vi "fake lock-in module.vi"(9 "Master mailbox":T6, 11 "Module mailbox":T6) -> ()   [LabVIEW 2024, in "Lock-in module.lvlib"]
uses:
  Lock-in module.lvlib
  Messenger service/Data types/Mailbox address.ctl
  ctl/ACQ status.ctl
  <instrlib>/Zurich Instruments LabOne/Public/ziTypeHandle.ctl
  <instrlib>/Zurich Instruments LabOne/Public/Modules/ziTypeModHandle.ctl
  ctl/ACQ info.ctl
  ctl/Mode.ctl
  Messenger service/Data types/Module name.ctl
  ctl/MFLI_message for module.ctl
  ctl/MFLI_command enum.ctl
  ctl/ACQ parameters.ctl
  ctl/MFLI_parameter and value.ctl
  ctl/MFLI_node.ctl
  <instrlib>/Zurich Instruments LabOne/Public/Data/ziTypeDemodSampleSingle.ctl
  <instrlib>/Zurich Instruments LabOne/Zurich Instruments LabOne.lvlib
  Messenger service/MessengerLib.lvlib
panel:
  out "Mode":T1=enum."Point"
  out "ACQ  status":T2={"Lock-in Handle"={"handleValid"=FALSE, "Conn"=0, "Path Prefix"="", "Handle"=0, "Connected"=FALSE, "Clockbase(s)"=0.0}, "Address"="DEV", "ModuleHandles"=[], "Lock-in info"={"In50"=FALSE, "InAC"=FALSE, "InDiff"=FALSE, "Out50"=FALSE, "OutEN"=FALSE, "OutF[Hz]"=0.0, "OutA[V]"=0.0, "DemEN"=FALSE, "Const[ms]"=0.0, "Order[-]"=0, "Phase [°]"=0.0}} {"ModuleHandles"."ModHandle" format="0x%08x"; "ModuleHandles"."Conn" format="0x%08x"; "Lock-in Handle"."Handle" format="0x%08x"; "Lock-in Handle"."Conn" format="0x%08x"}
  out "Selected Device":string
  out "Initialized":bool
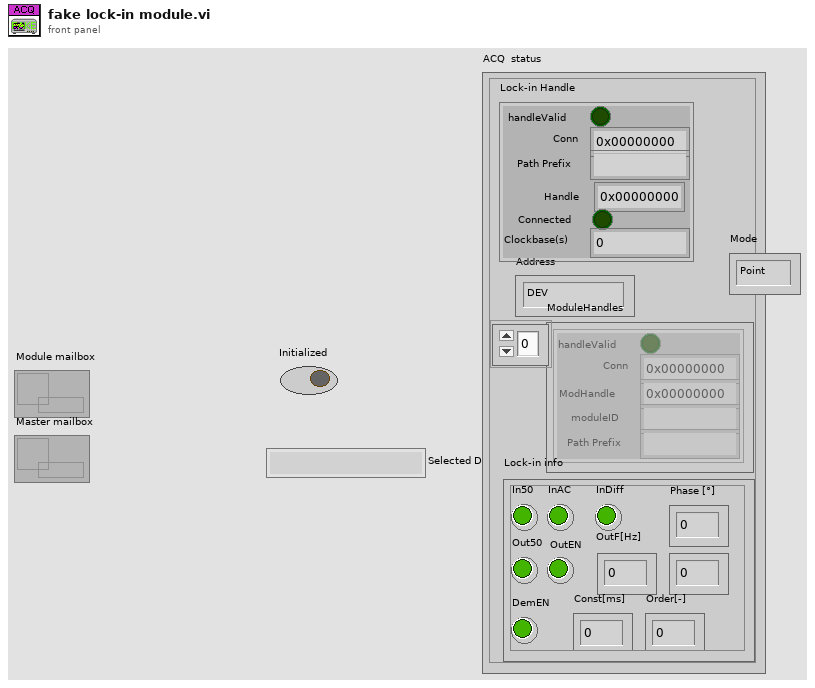
[diagram p1: front panel]
types:
  T1 = typedef "Lock-in module.lvlib/Mode.ctl" = enum16{"None", "Point", "Scope", "Both", "DAQ"}
  T2 = typedef "Lock-in module.lvlib/ACQ status.ctl" = cluster{"Lock-in Handle":T3, "Address":string, "ModuleHandles":T4[], "Lock-in info":T5}
  T3 = typedef "Zurich Instruments LabOne.lvlib/ziTypeHandle.ctl" = cluster{"handleValid":bool, "Conn":u64, "Path Prefix":string, "Handle":u64, "Connected":bool, "Clockbase(s)":dbl}
  T4 = typedef "Zurich Instruments LabOne.lvlib/ziTypeModHandle.ctl" = cluster{"handleValid":bool, "Conn":u64, "ModHandle":u64, "moduleID":string, "Path Prefix":string}
  T5 = typedef "Lock-in module.lvlib/ACQ info.ctl" = cluster{"In50":bool, "InAC":bool, "InDiff":bool, "Out50":bool, "OutEN":bool, "OutF[Hz]":dbl, "OutA[V]":dbl, "DemEN":bool, "Const[ms]":dbl, "Order[-]":i32, "Phase [°]":dbl}
  T6 = typedef "MessengerLib.lvlib/Mailbox address.ctl" = refnum<queue>
  T7 = typedef "Module name.ctl" = enum16{"Emty", "Magnet", "VTI", "Excitation", "Servo", "Acquisition", "Rotator", "Digitizer", "SMU2450", "Carousel", "Multimeter", "Tmp monitor", "Power monitor"}
  T8 = typedef "Lock-in module.lvlib/ACQ parameters.ctl" = cluster{"Filter order":dbl, "Time constant [ms]":dbl, "F_Mod [kHz]":dbl, "Amp_Mod [mV]":dbl, "Enable output":u16, "Phase [°]":dbl}
  T9 = typedef "Lock-in module.lvlib/MFLI_parameter and value.ctl" = cluster{"parameter":T10, "value":dbl}
  T10 = typedef "Lock-in module.lvlib/MFLI_node.ctl" = enum16{"None", "filter_order [-]", "filter_constant [ms]", "in_diff", "in_autorange", "in_imp50", "in_AC", "osc_freq [kHz]", "out_ampl [V]", "out_autorange", "out_imp50", "enable output", "enamble ampl", "scope_enable", "scope_rate", "scope_len", "scope_trigEn", "AuxOut_amplify", "Phase_deg", "AuxOut_select"}
  T11 = typedef "Zurich Instruments LabOne.lvlib/ziTypeDemodSampleSingle.ctl" = cluster{"Timestamps (ticks)":u64, "X (Vrms)":dbl, "Y (Vrms)":dbl, "Osc Phase (deg)":dbl, "Freq (Hz)":dbl, "DIO":u32, "AuxIn0 (V)":dbl, "AuxIn1 (V)":dbl, "Trigger":u32}
  T12 = typedef "Lock-in module.lvlib/MFLI_command enum.ctl" = enum16{"Initialize", "Update", "Set parameters", "Set module", "Set individual parameters", "Get point", "Get array", "Disconnect", "End", "Ignore"}
  T13 = typedef "Lock-in module.lvlib/MFLI_message for module.ctl" = cluster{"Command":T12, "Data":variant}
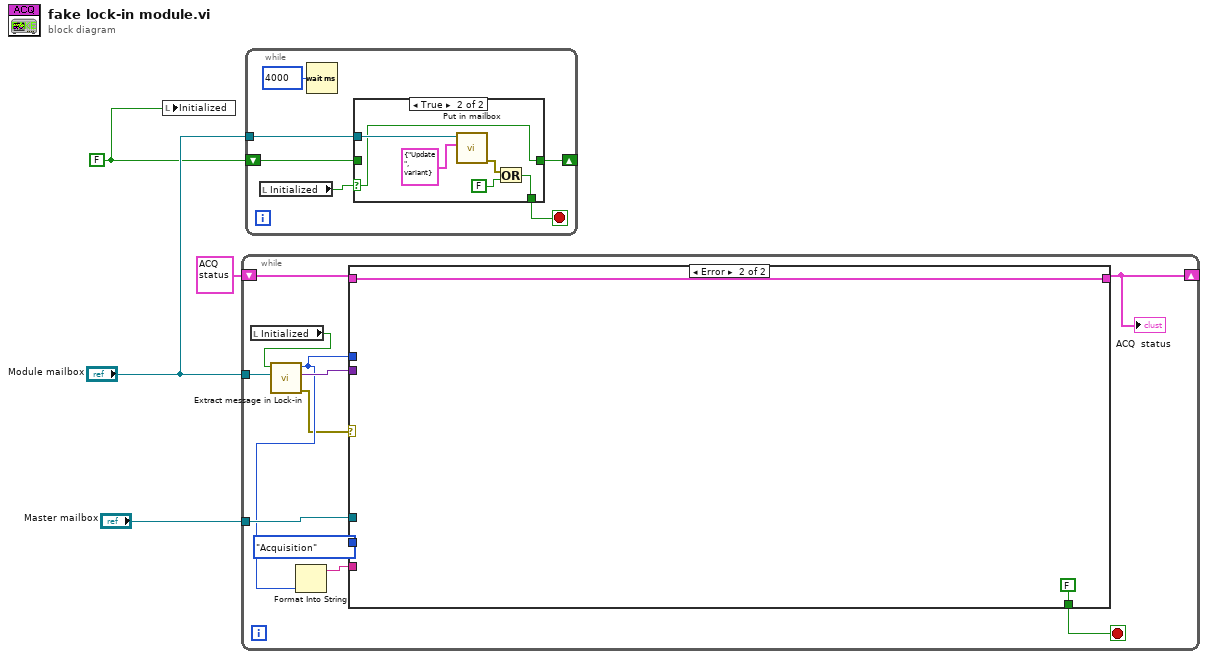
[diagram p0: block diagram]
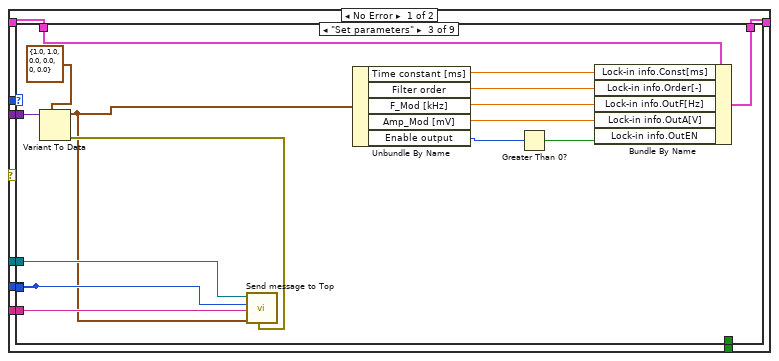
[diagram p2: hidden frame]
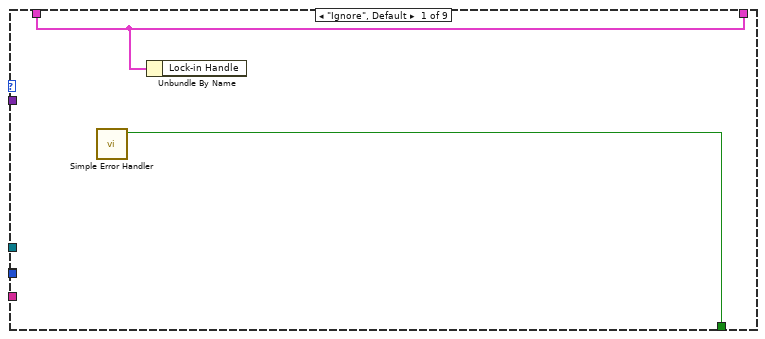
[diagram p3: hidden frame]
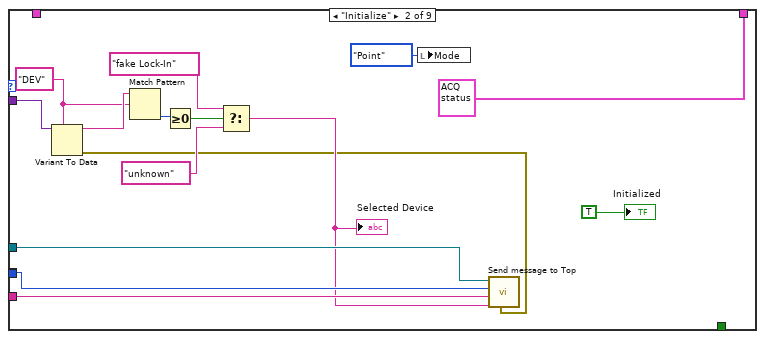
[diagram p4: hidden frame]
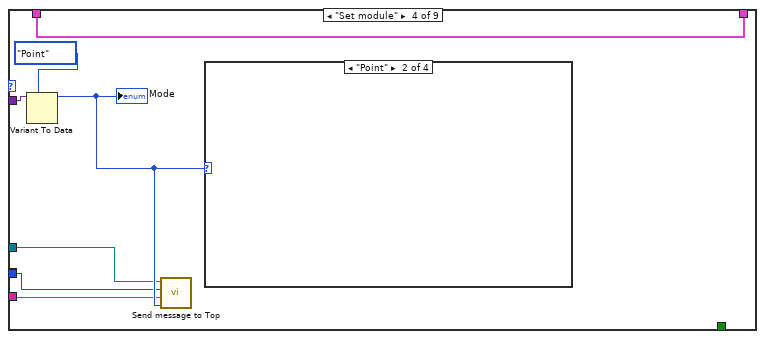
[diagram p5: hidden frame]
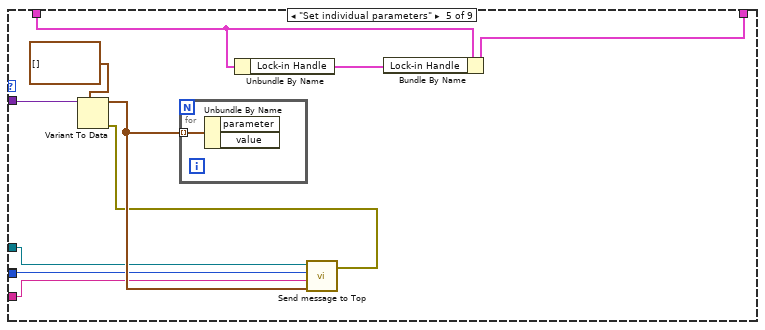
[diagram p9: hidden frame]
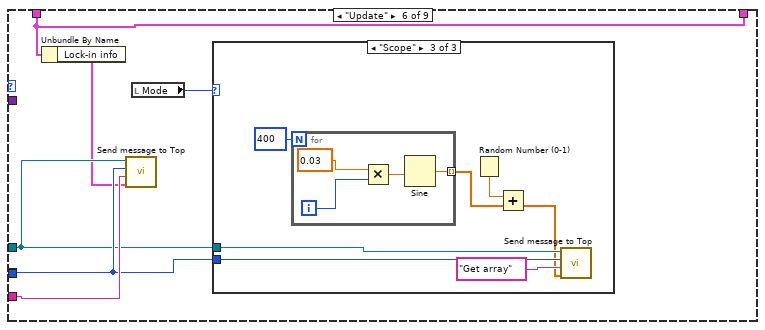
[diagram p10: hidden frame]
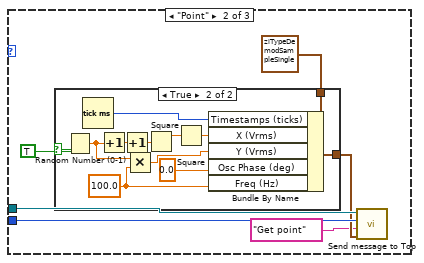
[diagram p12: hidden frame]
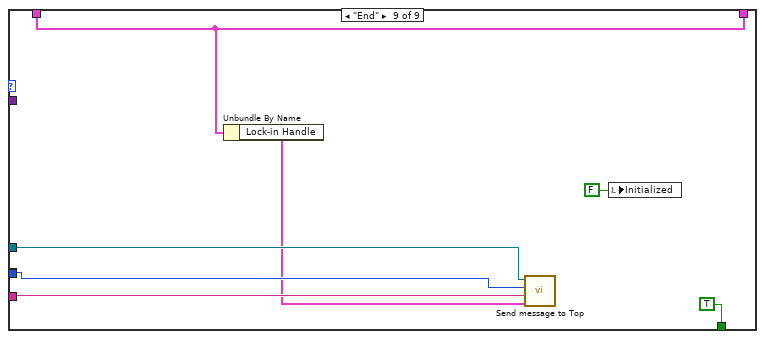
[diagram p16: hidden frame]
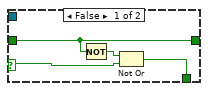
[diagram p17: hidden frame]
diagram:
  w1 = FALSE
  n1 = local write "Initialized"(w1) -> ()
  n2 = while {
    tunnel: "Module mailbox" -> [w15]
    tunnel: "Master mailbox" -> [w14]
    shift-right: [w11] -> _
    shift-left: T2 {"Lock-in Handle"={"handleValid"=FALSE, "Conn"=0, "Path Prefix"="", "Handle"=0, "Connected"=FALSE, "Clockbase(s)"=0.0}, "Address"="DEV", "ModuleHandles"=[], "Lock-in info"={"In50"=FALSE, "InAC"=FALSE, "InDiff"=FALSE, "Out50"=FALSE, "OutEN"=FALSE, "OutF[Hz]"=0.0, "OutA[V]"=0.0, "DemEN"=FALSE, "Const[ms]"=0.0, "Order[-]"=0, "Phase [°]"=0.0}} -> [w10]
    stop <- w12 stop-if-true
    n3 = local read "Initialized"() -> (w9:bool)
    n4 = call "Extract message in Lock-in.vi"("Module mailbox"=w15, "Initialized?"=w9) -> ("error out"=w5:errorcluster, "Data"=w13:variant, "Command out"=w7:T12)  [unwired: 7 in]
    n5 = Format Into String(w7) -> (resulting string=w8:string)  [unwired: 3 in, 1 out]
    n6 = case shown="Error" w5 {
      tunnel: w14 -> [w23 _]
      tunnel: w13 -> [w22 _]
      tunnel: [w21 FALSE ("error?")] -> w12
      tunnel: [w20 w119] -> w11
      tunnel: w10 -> [w19 w119]
      tunnel: w8 -> [w18 _]
      tunnel: w7 -> [w17 _]
      tunnel: Module_name."Acquisition" ("Module") -> [w16 _]
      frame No Error {
        n7 = case shown="\"Set parameters\"" w17 {
          tunnel: w23 -> [_ w39 w51 w56 w64 w76 _ _ w115]
          tunnel: w22 -> [_ w40 w55 w61 w72 _ _ _ _]
          tunnel: [w25 _ _ _ _ _ _ _ TRUE] -> w21
          tunnel: [w24 T2 {"Lock-in Handle"={"handleValid"=FALSE, "Conn"=0, "Path Prefix"="", "Handle"=0, "Connected"=FALSE, "Clockbase(s)"=0.0}, "Address"="DEV", "ModuleHandles"=[], "Lock-in info"={"In50"=FALSE, "InAC"=FALSE, "InDiff"=FALSE, "Out50"=FALSE, "OutEN"=FALSE, "OutF[Hz]"=0.0, "OutA[V]"=0.0, "DemEN"=FALSE, "Const[ms]"=0.0, "Order[-]"=0, "Phase [°]"=0.0}} w52 w62 w70 w75 w109 w110 w116] -> w20
          tunnel: w19 -> [w24 _ w53 w62 w69 w75 w109 w110 w116]
          tunnel: w18 -> [_ w38 w50 w58 w66 w78 _ _ w112]
          tunnel: w16 -> [_ w37 w49 _ w65 w77 _ _ w113]
          tunnel: w16 -> [_ _ _ w57 _ _ _ _ _]
          frame "Ignore", Default {
            n8 = call <vilib>:"Simple Error Handler.vi"() -> ("error?"=w25:bool)  [unwired: 5 in, 4 out]
            n9 = Unbundle By Name(w24) -> ()  [unwired: 1 out]
          }
          frame "Initialize" {
            w35 = "DEV" ("Address")
            n10 = Variant To Data(type=w35, Variant=w40) -> (data=w36:string, error out=w29:errorcluster)  [unwired: 1 in]
            n11 = Match Pattern(string=w36, regular expression=w35) -> (offset past match=w34:i32)  [unwired: 1 in, 3 out]
            n12 = Greater Or Equal To 0?(x=w34) -> (x >= 0?=w28:bool)
            n13 = Select(t="fake Lock-In" ("Address"), s=w28, f="unknown" ("Address")) -> (s? t:f=w31:string)
            "Selected Device" <- w31
            n14 = local write "Mode"(Mode."Point" ("Mode")) -> ()
            n15 = call "Send message to Top.vi"("Error in (no error)"=w29, "Data"=w31, "Response"=w38, "Module"=w37, "Mailbox address in"=w39) -> ()  [unwired: 5 in, 2 out]
            "Initialized" <- TRUE ("Initialized")
          }
          frame "Set parameters" {
            n16 = Variant To Data(type=T8 {"Filter order"=1.0, "Time constant [ms]"=1.0, "F_Mod [kHz]"=0.0, "Amp_Mod [mV]"=0.0, "Enable output"=0, "Phase [°]"=0.0} ("ACQ parameters"), Variant=w55) -> (data=w47:T8, error out=w48:errorcluster)  [unwired: 1 in]
            n17 = call "Send message to Top.vi"("Error in (no error)"=w48, "Data"=w47, "Response"=w50, "Module"=w49, "Mailbox address in"=w51) -> ()  [unwired: 5 in, 2 out]
            n18 = Unbundle By Name(w47) -> ("Time constant [ms]"=w46:dbl, "Filter order"=w45:dbl, "F_Mod [kHz]"=w41:dbl, "Amp_Mod [mV]"=w42:dbl, "Enable output"=w44:u16)
            n19 = Greater Than 0?(x=w44) -> (x > 0?=w43:bool)
            n20 = Bundle By Name(cluster=w53, "Lock-in info.Const[ms]"=w46, "Lock-in info.Order[-]"=w45, "Lock-in info.OutF[Hz]"=w41, "Lock-in info.OutA[V]"=w42, "Lock-in info.OutEN"=w43) -> (w52:T2)
          }
          frame "Set module" {
            n21 = Variant To Data(type=Mode."Point" ("Mode"), Variant=w61) -> (data=w59:T1)  [unwired: 1 in, 1 out]
            "Mode" <- w59
            n22 = call "Send message to Top.vi"("Data"=w59, "Response"=w58, "Module"=w57, "Mailbox address in"=w56) -> ()  [unwired: 6 in, 2 out]
            n23 = case shown="\"Point\"" w59 {
              frame "None", Default {
              }
              frame "Point" {
              }
              frame "Scope" {
              }
              frame "Both" {
              }
            }
          }
          frame "Set individual parameters" {
            n24 = Variant To Data(type=T9[] [] ("Array"), Variant=w72) -> (data=w67:T9[], error out=w63:errorcluster)  [unwired: 1 in]
            n25 = for {
              tunnel: w67 -> [w73] mode=indexing
              n26 = Unbundle By Name(w73) -> ()  [unwired: 2 out]
            }
            n27 = Unbundle By Name(w69) -> ("Lock-in Handle"=w68:T3)
            n28 = call "Send message to Top.vi"("Error in (no error)"=w63, "Data"=w67, "Response"=w66, "Module"=w65, "Mailbox address in"=w64) -> ()  [unwired: 5 in, 2 out]
            n29 = Bundle By Name(cluster=w69, "Lock-in Handle"=w68) -> (w70:T2)
          }
          frame "Update" {
            n30 = Unbundle By Name(w75) -> ("Lock-in info"=w74:T5)
            n31 = call "Send message to Top.vi"("Data"=w74, "Response"=w78, "Module"=w77, "Mailbox address in"=w76) -> ()  [unwired: 6 in, 2 out]
            n32 = local read "Mode"() -> (w79:T1)
            n33 = case shown="\"Scope\"" w79 {
              tunnel: w76 -> [_ w85 w104]
              tunnel: w77 -> [_ w84 w103]
              frame "None", Default {
              }
              frame "Point" {
                n34 = case shown="True" TRUE {
                  tunnel: T11 {"Timestamps (ticks)"=0, "X (Vrms)"=0.0, "Y (Vrms)"=0.0, "Osc Phase (deg)"=0.0, "Freq (Hz)"=0.0, "DIO"=0, "AuxIn0 (V)"=0.0, "AuxIn1 (V)"=0.0, "Trigger"=0} ("Update data") -> [w86 w97]
                  tunnel: [w86 w95] -> w82
                  frame False {
                  }
                  frame True {
                    w91 = 100.0 ("Freq (Hz)")
                    n35 = Random Number (0-1)() -> (number: 0 to 1=w90:dbl)
                    n36 = Tick Count (ms)() -> (millisecond timer value=w96:u32)
                    n37 = Increment(x=w90) -> (x+1=w89:dbl)
                    n38 = Increment(x=w89) -> (x+1=w87:dbl)
                    n39 = Multiply(x=w90, y=w91) -> (x*y=w92:dbl)
                    n40 = Square(x=w87) -> (x^2=w88:dbl)
                    n41 = Square(x=w88) -> (x^2=w93:dbl)
                    n42 = Bundle By Name(cluster=w97, "Timestamps (ticks)"=w96, "X (Vrms)"=w93, "Y (Vrms)"=w92, "Osc Phase (deg)"=0.0, "Freq (Hz)"=w91) -> (w95:T11)
                  }
                }
                n43 = call "Send message to Top.vi"("Data"=w82, "Response"="Get point", "Module"=w84, "Mailbox address in"=w85) -> ()  [unwired: 6 in, 2 out]
              }
              frame "Scope" {
                n44 = for {
                  N: 400 -> [_]
                  tunnel: [w108] -> w100 mode=indexing
                  i -> [w106]
                  n45 = Multiply(x=0.03, y=w106) -> (x*y=w107:dbl)
                  n46 = Sine(x=w107) -> (sin(x)=w108:dbl)
                }
                n47 = Random Number (0-1)() -> (number: 0 to 1=w98:dbl)
                n48 = Add(x=w98, y=w100) -> (x+y=w99:dbl[])
                n49 = call "Send message to Top.vi"("Data"=w99, "Response"="Get array", "Module"=w103, "Mailbox address in"=w104) -> ()  [unwired: 6 in, 2 out]
              }
            }
          }
          frame "Get point" {
          }
          frame "Get array" {
          }
          frame "End" {
            n50 = Unbundle By Name(w116) -> ("Lock-in Handle"=w111:T3)
            n51 = call "Send message to Top.vi"("Data"=w111, "Response"=w112, "Module"=w113, "Mailbox address in"=w115) -> ()  [unwired: 6 in, 2 out]
            n52 = local write "Initialized"(FALSE ("Initialized")) -> ()
          }
        }
      }
      frame Error {
      }
    }
    "ACQ  status" <- w11
  }
  n53 = while {
    tunnel: "Module mailbox" -> [w124]
    shift-right: [w122] -> _
    shift-left: w1 -> [w121]
    stop <- w123 stop-if-true
    n54 = local read "Initialized"() -> (w120:bool)
    n55 = Wait (ms)(milliseconds to wait=u32 4000) -> ()  [unwired: 1 out]
    n56 = case shown="True" w120 {
      selector: w120 -> [w127 w130]
      tunnel: w124 -> [_ w135]
      tunnel: [w126 w131] -> w123
      tunnel: w121 -> [w129 _]
      tunnel: [w129 w130] -> w122
      frame False {
        n57 = Not(x=w129) -> (.not. x?=w128:bool)
        n58 = Not Or(1:w127, 2:w128) -> (0:w126:bool)
      }
      frame True {
        n59 = call "Put in mailbox.vi"("Message"=T13 {"Command"=enum."Update", "Data"=variant} ("MSG for  ACQ"), "Queue in"=w135) -> ("error out"=w133:errorcluster)  [unwired: 7 in, 2 out]
        n60 = Or(x=w133, y=FALSE) -> (x .or. y?=w131:bool)
      }
    }
  }
